vi "EventStreamToDecayCurve.vi"(8 "Error In":errorcluster, 10 "EventData":u16[](array[numeric]) format="%04x", 11 "MT-OverflowsStart":u64) -> (0 "Error Out":errorcluster, 1 "PhotonCount":u64, 2 "DecaySum":u32[](array[numeric]), 3 "MT-Overflows":u64, 4 "EventMT":u32[](array[numeric]), 5 "PhotInfo64":T1[](array[typedef]) {"flags" max=3 format="%016b"; "rout_chan" step=1; "micro_time" step=1; "mtime" step=1})   [LabVIEW 2019]
doc: "This VI goes through an EventData-Array received from 'SPC_read_fifo.vi' and interprets the events as markers or photons and populates a single decay curve according to their microTime value.\n<b>Note:</b> Events are always 2 word wide, and received in reversed byte and word order.\n\ninfo@becker-hickl.com"
uses:
  SPC_Controls/SPC_PhotInfo64.ctl
panel:
  out "Event":u32 format="%08x"
  out "GAPs":u64[](array[numeric])
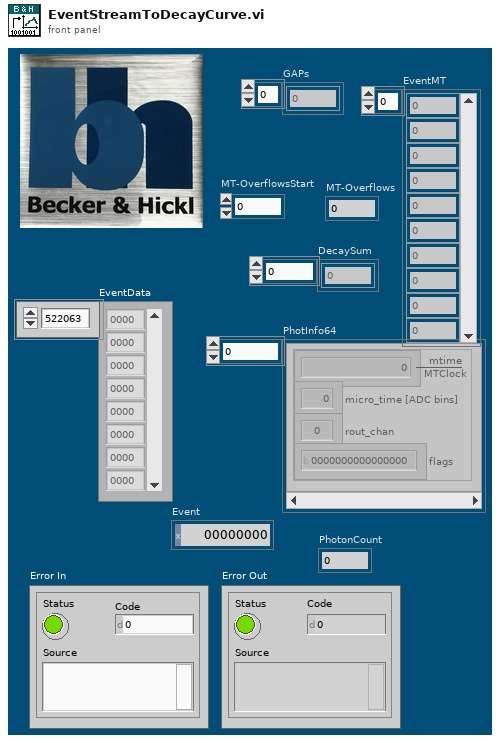
[diagram p1: front panel]
types:
  T1 = typedef "SPC_PhotInfo64.ctl" = cluster{"mtime":u64, "micro_time":u16, "rout_chan":u16, "flags":u16}
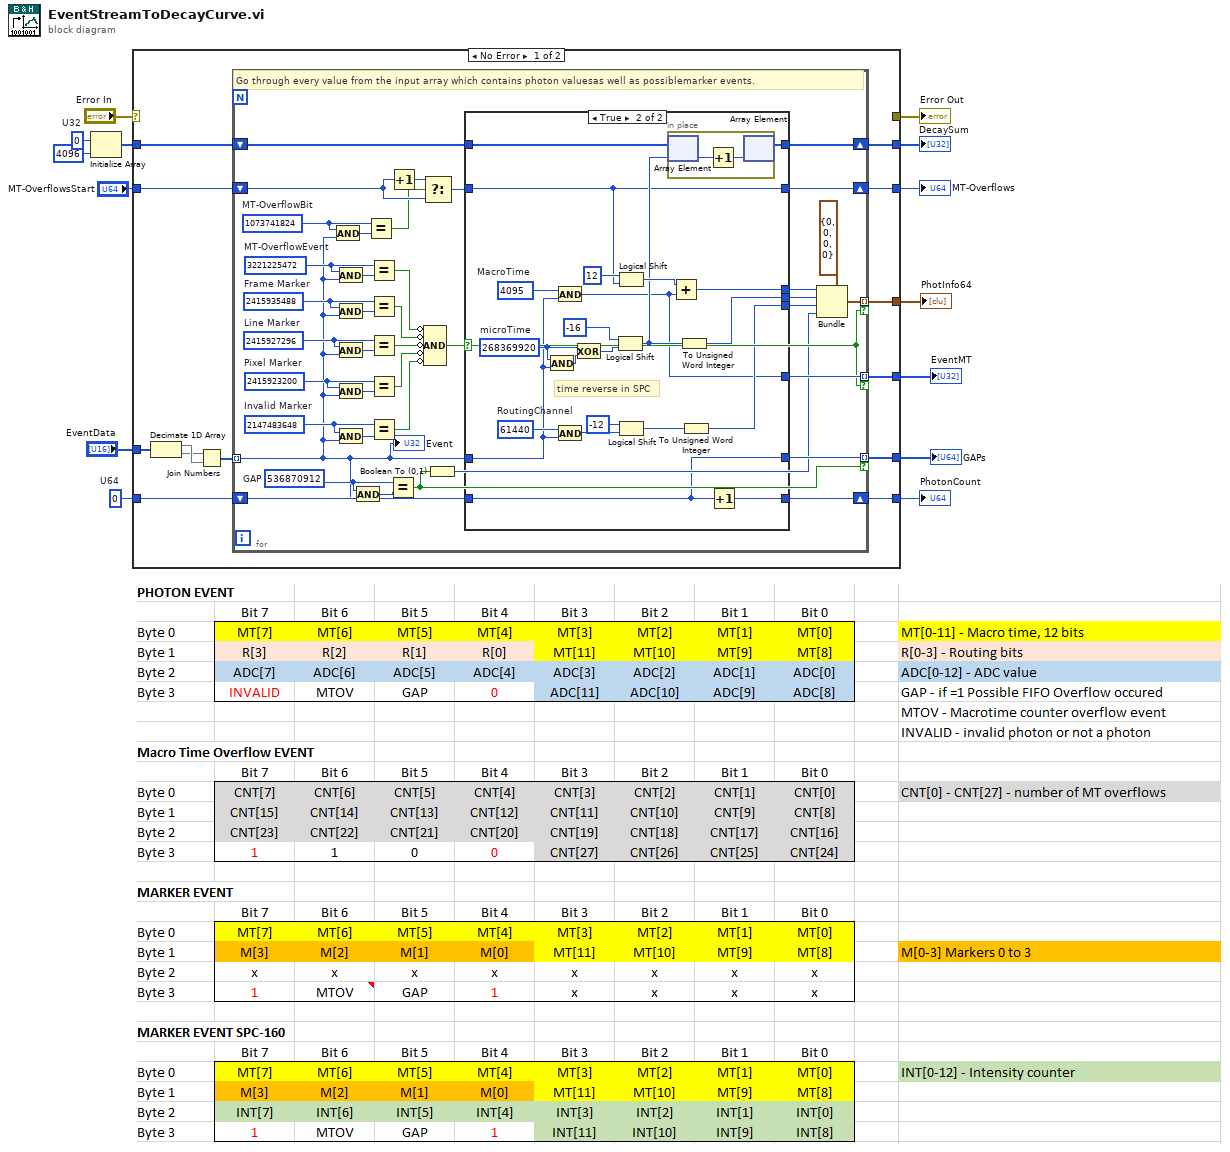
[diagram p0: block diagram]
diagram:
  w4 = u64 0  # U64
  w10 = u32 0  # U32
  n1 = Initialize Array(w10, 4096 ("dimension size")) -> (w9:u32[])
  n2 = case shown="No Error" "Error In" {
    selector: "Error In" -> [_ w94]
    tunnel: [_ w94] -> w13
    tunnel: "EventData" -> [w27 _]
    tunnel: [w26 _] -> w11
    tunnel: w9 -> [w25 _]
    tunnel: w4 -> [w17 _]
    tunnel: [w21 _] -> w3
    tunnel: "MT-OverflowsStart" -> [w20 _]
    tunnel: [w19 _] -> w6
    tunnel: [w18 _] -> w5
    tunnel: [w16 _] -> w2
    tunnel: [w15 _] -> w1
    frame No Error {
      n3 = Decimate 1D Array(w27) -> (w23:u16[], w22:u16[])
      n4 = Join Numbers(hi=w22, lo=w23) -> ((hi.lo)=w24:u32[])
      n5 = for {
        tunnel: w24 -> [w31] mode=indexing
        shift-right: [w56] -> w21
        shift-left: w17 -> [w55]
        shift-right: [w63] -> w26
        shift-left: w25 -> [w64]
        shift-right: [w51] -> w19
        shift-left: w20 -> [w38]
        tunnel: [w48] -> w18 mode=indexing if=w35
        tunnel: [w36] -> w16 mode=indexing if=w35
        tunnel: [w34] -> w15 mode=indexing if=w30
        w32 = u32 536870912  # GAP
        w41 = u32 1073741824  # MT-OverflowBit
        w42 = u32 2147483648  # Invalid Marker
        w58 = u32 2415923200  # Pixel Marker
        w60 = u32 2415927296  # Line Marker
        w43 = u32 3221225472  # MT-OverflowEvent
        w66 = u32 2415935488  # Frame Marker
        # "Go through every value from the input array which contains photon valuesas well as possiblemarker events."
        n6 = And(x=w41, y=w31) -> (x .and. y?=w40:u32)
        n7 = And(x=w43, y=w31) -> (x .and. y?=w62:u32)
        n8 = And(x=w66, y=w31) -> (x .and. y?=w65:u32)
        n9 = And(x=w60, y=w31) -> (x .and. y?=w61:u32)
        n10 = And(x=w58, y=w31) -> (x .and. y?=w59:u32)
        n11 = And(x=w42, y=w31) -> (x .and. y?=w57:u32)
        n12 = And(x=w32, y=w31) -> (x .and. y?=w33:u32)
        n13 = Equal?(x=w41, y=w40) -> (x = y?=w28:bool)
        n14 = Equal?(x=w43, y=w62) -> (x = y?=w50:bool)
        n15 = Equal?(x=w66, y=w65) -> (x = y?=w54:bool)
        n16 = Equal?(x=w60, y=w61) -> (x = y?=w53:bool)
        n17 = Equal?(x=w58, y=w59) -> (x = y?=w52:bool)
        n18 = Equal?(x=w42, y=w57) -> (x = y?=w44:bool)
        n19 = Equal?(x=w32, y=w33) -> (x = y?=w30:bool)
        n20 = Increment(x=w38) -> (x+1=w39:u64)
        n21 = Select(t=w39, s=w28, f=w38) -> (s? t:f=w37:u64)
        n22 = Compound Arithmetic op=AND(invert w50, invert w54, invert w53, invert w52, invert w44) -> (w35:bool)
        n23 = Boolean To (0,1)(Boolean=w30) -> (0, 1=w29:i16)
        n24 = case shown="True" w35 {
          tunnel: w55 -> [w68 w70]
          tunnel: w31 -> [_ w71]
          tunnel: w64 -> [w69 w90]
          tunnel: [w69 w91] -> w63
          tunnel: [w68 w74] -> w56
          tunnel: w37 -> [w67 w73]
          tunnel: [w67 w73] -> w51
          tunnel: [_ w81] -> w49
          tunnel: [_ w78] -> w47
          tunnel: [_ w77] -> w46
          tunnel: [_ w72] -> w36
          tunnel: [_ w70] -> w34
          frame False {
          }
          frame True {
            w83 = u32 4095  # MacroTime
            w88 = u32 61440  # RoutingChannel
            w89 = u32 268369920  # microTime
            # "time reverse in SPC"
            n25 = And(x=w89, y=w71) -> (x .and. y?=w76:u32)
            n26 = And(x=w83, y=w71) -> (x .and. y?=w72:u32)
            n27 = And(x=w88, y=w71) -> (x .and. y?=w87:u32)
            n28 = Exclusive Or(1:w76, 2:w89) -> (0:w75:u32)
            n29 = Logical Shift(y=-16, x=w75) -> (x << y=w80:u32)
            n30 = Logical Shift(y=i16 12, x=w73) -> (x << y=w82:u64)
            n31 = Logical Shift(y=i16 -12, x=w87) -> (x << y=w79:u32)
            n32 = in-place {
              n33 = in-place-array #1(w90, w80) -> (w93:u32)
              n34 = Increment(x=w93) -> (x+1=w92:u32)
              n35 = in-place-array #1(w92) -> (w91:u32[])  [unwired: 1 out]
            }
            n36 = Add(x=w82, y=w72) -> (x+y=w81:u64)
            n37 = To Unsigned Word Integer(number=w80) -> (unsigned 16bit integer=w78:u16)
            n38 = To Unsigned Word Integer(number=w79) -> (unsigned 16bit integer=w77:u16)
            n39 = Increment(x=w70) -> (x+1=w74:u64)
          }
        }
        n40 = Bundle(cluster=T1 {"mtime"=0, "micro_time"=0, "rout_chan"=0, "flags"=0} ("SPC_PhotInfo"), "mtime"=w49, "micro_time"=w47, "rout_chan"=w46, "flags"=w29) -> (w48:T1)
        "Event" <- w31
      }
    }
    frame Error {
    }
  }
  "Error Out" <- w13
  "DecaySum" <- w11
  "PhotonCount" <- w3
  "MT-Overflows" <- w6
  "PhotInfo64" <- w5
  "EventMT" <- w2
  "GAPs" <- w1
